vi "DelayPhase.vi"(7 "Use fixed delay":bool, 9 "fixed cos_fi":fxp<+/-,16,0>, 10 "fixed sin fi":fxp<+/-,16,0>, 11 "delay phase":fxp<+,64,64>) -> (2 "cos_fi":fxp<+/-,16,0>, 3 "sin fi":fxp<+/-,16,0>)   [LabVIEW 2013]
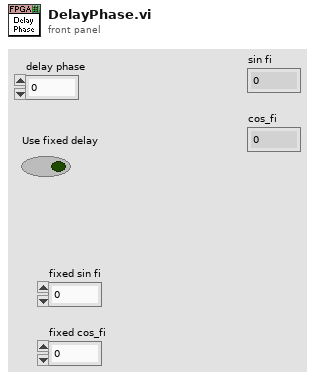
[diagram p1: front panel]
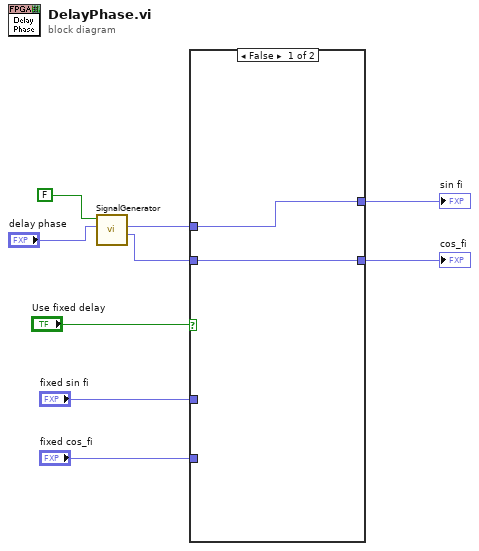
[diagram p0: block diagram]
diagram:
  n1 = call "SignalGenerator.vi"("phase"="delay phase", "Reset"=FALSE) -> ("Cos"=w1:fxp<+/-,16,0>, "Sin"=w2:fxp<+/-,16,0>)  [unwired: 7 in, 1 out]
  n2 = case shown="False" "Use fixed delay" {
    tunnel: [w11 w13] -> w6
    tunnel: "fixed sin fi" -> [_ w13]
    tunnel: [w10 w12] -> w4
    tunnel: "fixed cos_fi" -> [_ w12]
    tunnel: w2 -> [w11 _]
    tunnel: w1 -> [w10 _]
    frame False {
    }
    frame True {
    }
  }
  "sin fi" <- w6
  "cos_fi" <- w4
